vi "System Restore.vi"(0 "Instrument Handle In":i32, 2 "State":u16 caption="Number", 3 "error in":errorcluster) -> (6 "Instrument Handle Out":i32, 9 "error out":errorcluster)   [LabVIEW 8.6, in "ZTScopeM.lvlib"]
doc: "Configure the instrument boot location."
uses:
  ZTScopeM.lvlib
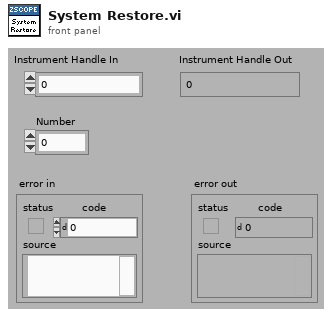
[diagram p1: front panel]
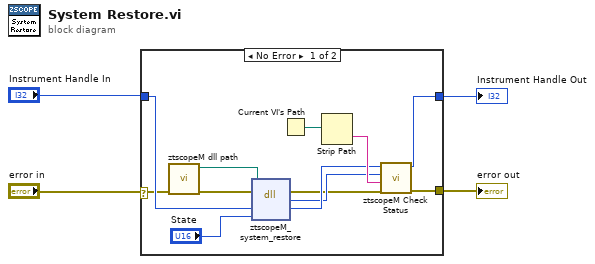
[diagram p0: block diagram]
diagram:
  n1 = case shown="No Error" "error in" {
    selector: "error in" -> [w8 w17]
    tunnel: [w11 w17] -> w2
    tunnel: "Instrument Handle In" -> [w16 w18]
    tunnel: [w10 w18] -> w3
    frame #0 {
      n2 = call "ztscopeM dll path.vi"("error in (no error)"=w8) -> ("error out"=w6:errorcluster, "<instrument>.dll path"=w7:path)  [unwired: 9 in]
      n3 = dll-call lib="C:/Program Files (x86)/National Instruments/LabVIEW 2013/instr.lib/ztscopem/ztscopeM.dll" fn="ztscopeM_system_restore"(path in=w7, error in=w6, "instrumentHandle"=w16, "Number"="State") -> (error out=w5:errorcluster, w12:i32, "instrumentHandle"=w13:i32)  [unwired: 2 in, 1 out]
      n4 = Current VI's Path() -> (path=w15:path)
      n5 = Strip Path(path=w15) -> (name=w14:string)  [unwired: 1 out]
      n6 = call "ztscopeM Check Status.vi"("error in"=w5, "name of VI"=w14, "status (return code)"=w12, "instrument handle in"=w13) -> ("error out"=w11:errorcluster, "instrument handle out"=w10:i32)  [unwired: 2 in]
    }
    frame #1 {
    }
  }
  "Instrument Handle Out" <- w3
  "error out" <- w2
